vi "Win Msg Q Size.vi"(4 "error in (no error)":errorcluster, 7 "win msg queue":T1) -> (0 "error out":errorcluster, 1 "Items in queue":i32, 3 "win msg queue out":T1)   [LabVIEW 2011]
doc: "Returns the number of messages waiting in the queue specified by win msg queue.\n\nErrors:\n6751: not a valid windows message queue."
uses:
  Win Msg Q RefNum.ctl
  lvwinmsg.dll
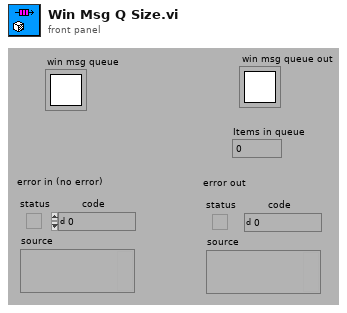
[diagram p1: front panel]
types:
  T1 = typedef "Win Msg Q RefNum.ctl" = refnum<k1>
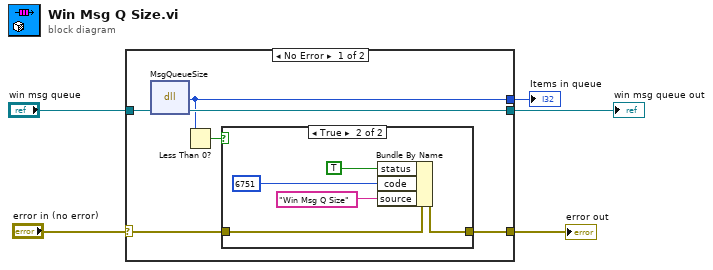
[diagram p0: block diagram]
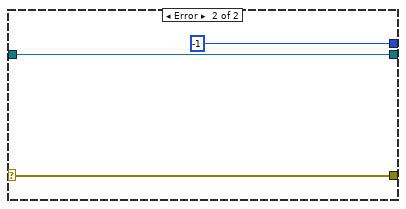
[diagram p3: hidden frame]
diagram:
  n1 = case shown="No Error" "error in (no error)" {
    selector: "error in (no error)" -> [w6 w18]
    tunnel: "win msg queue" -> [w11 w20]
    tunnel: [w9 -1] -> w2
    tunnel: [w7 w18] -> w4
    tunnel: [w10 w20] -> w3
    frame No Error {
      n2 = dll-call lib="C:/Development/SI.LIB/WIN32/WinMSGQ/lvwinmsg.dll" fn="MsgQueueSize"("win msg queue"=w11) -> (w9:i32, "win msg queue"=w10:T1)  [unwired: 3 in, 2 out]
      n3 = Less Than 0?(x=w9) -> (x < 0?=w8:bool)
      n4 = case shown="True" w8 {
        tunnel: [w12 w13] -> w7
        tunnel: w6 -> [w12 w14]
        frame False {
        }
        frame True {
          n5 = Bundle By Name(cluster=w14, "status"=TRUE, "code"=6751 ("Error Code"), "source"="Win Msg Q Size") -> (w13:errorcluster)
        }
      }
    }
    frame Error {
    }
  }
  "error out" <- w4
  "win msg queue out" <- w3
  "Items in queue" <- w2
